vi "PWM.vi"() -> ()   [LabVIEW 2019]
uses:
  <vilib>/myRIO/Instrument Drivers/Onboard IO/PWM/typedefs/PWM Reference.ctl
  <vilib>/myRIO/Common/Instrument Driver Framework/Utilities/typedefs/myRIO Generic Hardware Reference.ctl
  <vilib>/myRIO/Common/Instrument Driver Framework/Utilities/typedefs/Hardware Version Enum.ctl
  <vilib>/myRIO/Common/Instrument Driver Framework/Utilities/typedefs/myRIO v1.0 Reference.ctl
  <vilib>/myRIO/Common/Instrument Driver Framework/Utilities/typedefs/Generic FPGA Reference.ctl
  <vilib>/myRIO/Common/Instrument Driver Framework/myRIO v1.0/PWM/typedefs/PWM Channels Enum.ctl
  <vilib>/myRIO/Instrument Drivers/Onboard IO/PWM/typedefs/PWM Configuration.ctl
  <vilib>/userdefined/High Color/nirio_resource_hc.ctl
  <vilib>/myRIO/Instrument Drivers/Onboard IO/DI Block/typedefs/DI Block Reference.ctl
  <vilib>/myRIO/Common/Instrument Driver Framework/myRIO v1.0/DI Block/typedefs/DI Block Channels List.ctl
  <vilib>/myRIO/Common/Instrument Driver Framework/myRIO v1.0/DI Block/typedefs/DI Block Channels Enum.ctl
  <vilib>/myRIO/Common/Instrument Driver Framework/ELVIS III v1.0/DI Block/vis/ELVIS III v1.1 Open DI (N Samples).vi
  <vilib>/myRIO/Common/Instrument Driver Framework/Utilities/vis/Validate Channels.vi
  <vilib>/myRIO/Common/Instrument Driver Framework/ELVIS III v1.0/Resource Manager/vis/ELVIS III v1.0 Check For Different Banks.vi
  <vilib>/myRIO/Common/Instrument Driver Framework/ELVIS III v1.0/DI Block/vis/ELVIS III v1.0 DI Block Read.vi
  <vilib>/myRIO/Common/Instrument Driver Framework/ELVIS III v1.0/DI Block/vis/ELVIS III v1.0 Close DI Block.vi
  <vilib>/myRIO/Common/Instrument Driver Framework/myRIO v1.0/UART/vis/myRIO v1.0 Close UART.vi
  <vilib>/myRIO/Common/Instrument Driver Framework/Utilities/vis/Sample Rate To Ticks.vi
  <vilib>/myRIO/Common/Instrument Driver Framework/ELVIS III v1.0/DI Block/vis/ELVIS III v1.0 Unreserve DI Block.vi
  <vilib>/myRIO/Common/Instrument Driver Framework/ELVIS III v1.0/Resource Manager/vis/ELVIS III v1.0 Create Configuration List.vi
  <vilib>/myRIO/Common/Instrument Driver Framework/ELVIS III v1.0/DI Block/vis/ELVIS III v1.0 Build MUX Configuration DI Block.vi
  <vilib>/Utility/VariantDataType/GetNumericInfo.vi
  <vilib>/Utility/error.llb/Error Cluster From Error Code.vi
  <vilib>/myRIO/Common/Instrument Driver Framework/ELVIS III v1.0/ELVIS III v1.1 Open.vi
  <vilib>/myRIO/Common/Instrument Driver Framework/ELVIS III v1.0/Resource Manager/vis/ELVIS III v1.0 Reserve Channel List.vi
  <vilib>/myRIO/Common/Instrument Driver Framework/ELVIS III v1.0/Resource Manager/vis/ELVIS III v1.0 Configure IO.vi
  <vilib>/myRIO/Common/Instrument Driver Framework/myRIO v1.0/myRIO v1.0 Close.vi
  <vilib>/myRIO/Common/Instrument Driver Framework/ELVIS III v1.0/DI Block/vis/ELVIS III v1.0 Reserve DI Block.vi
  <vilib>/myRIO/Common/Instrument Driver Framework/ELVIS III v1.0/Resource Manager/vis/ELVIS III v1.0 Configure DMAs.vi
  <vilib>/myRIO/Common/Instrument Driver Framework/myRIO v1.0/Resource Manager/vis/myRIO v1.0 Block Write Configuration.vi
  <vilib>/myRIO/Common/Instrument Driver Framework/ELVIS III v1.0/DI Block/vis/ELVIS III v1.0 DI Block Read Bank B.vi
  <vilib>/myRIO/Common/Instrument Driver Framework/ELVIS III v1.0/DI Block/vis/ELVIS III v1.0 DI Block Read Bank A.vi
  <vilib>/Waveform/DWDTOps.llb/DWDT Boolean Array to Digital.vi
  <vilib>/myRIO/Common/Instrument Driver Framework/ELVIS III v1.0/Resource Manager/vis/ELVIS III v1.0 Unreserve Channel List.vi
  <vilib>/myRIO/Common/Instrument Driver Framework/ELVIS III v1.0/Resource Manager/vis/ELVIS III v1.0 Configure DI Mode.vi
  <vilib>/myRIO/Common/Instrument Driver Framework/Utilities/vis/FPGA Ref Manager.vi
  <vilib>/myRIO/Common/Instrument Driver Framework/ELVIS III v1.0/ELVIS III v1.0 Reset FPGA.vi
  <vilib>/myRIO/Common/Instrument Driver Framework/myRIO v1.0/IRQ/vis/myRIO v1.0 IRQ Info FGV.vi
  <vilib>/myRIO/Common/Instrument Driver Framework/myRIO v1.0/IRQ/vis/myRIO v1.0 Timer IRQ Info FGV.vi
  <vilib>/myRIO/Common/Instrument Driver Framework/myRIO v1.0/IRQ/vis/myRIO v1.0 ISR Agent.vi
  <vilib>/myRIO/Instrument Drivers/Utilities/vis/Reset Index.vi
  <vilib>/myRIO/Common/Instrument Driver Framework/myRIO v1.0/Resource Manager/vis/myRIO v1.0 Block Write Resource Manager.vi
  <vilib>/myRIO/Instrument Drivers/Onboard IO/PWM/vis/myRIO PWM Open.xnode
  <vilib>/myRIO/Instrument Drivers/Onboard IO/DI Block/vis/myRIO DI N Samples Open.xnode
  <vilib>/myRIO/Instrument Drivers/Utilities/Utilities.lvlib
  <vilib>/myRIO/Instrument Drivers/Onboard IO/PWM/PWM.lvlib
  <vilib>/myRIO/Instrument Drivers/Onboard IO/DI Block/DI Block.lvlib
panel:
  out "PWM Signal":digitalwaveform(graph)={"t0"=timestamp(0 s since 1904-01-01), "dt"=0.0001, "Y"={"transitions"=[], "data"=[]}}
  in  "Frequency [Hz]":dbl(knob)=500.0 min=40.0 max=1000.0 scale=40.0..1000.0
  in  "Duty Cycle":dbl(knob)=0.5 min=0.0 max=1.0 scale=0.0..1.0
  in  "?":bool
  # "ELVIS III Control IO"
  # "PWM"
  # "Overview: Generates a PWM signal on Bank A, Channel DIO0 (A/DIO0) with a set duty cycle and frequency and reads the signal on Bank A, Channel DIO1 (A/DIO1).\nInstructions:\n1. Connect A/DIO0 to A/DIO1 to read back the signal on the PWM Signal graph.\n2. Run the VI.\n3. Modify Duty Cycle or Frequency while the VI is running to change the PWM signal."
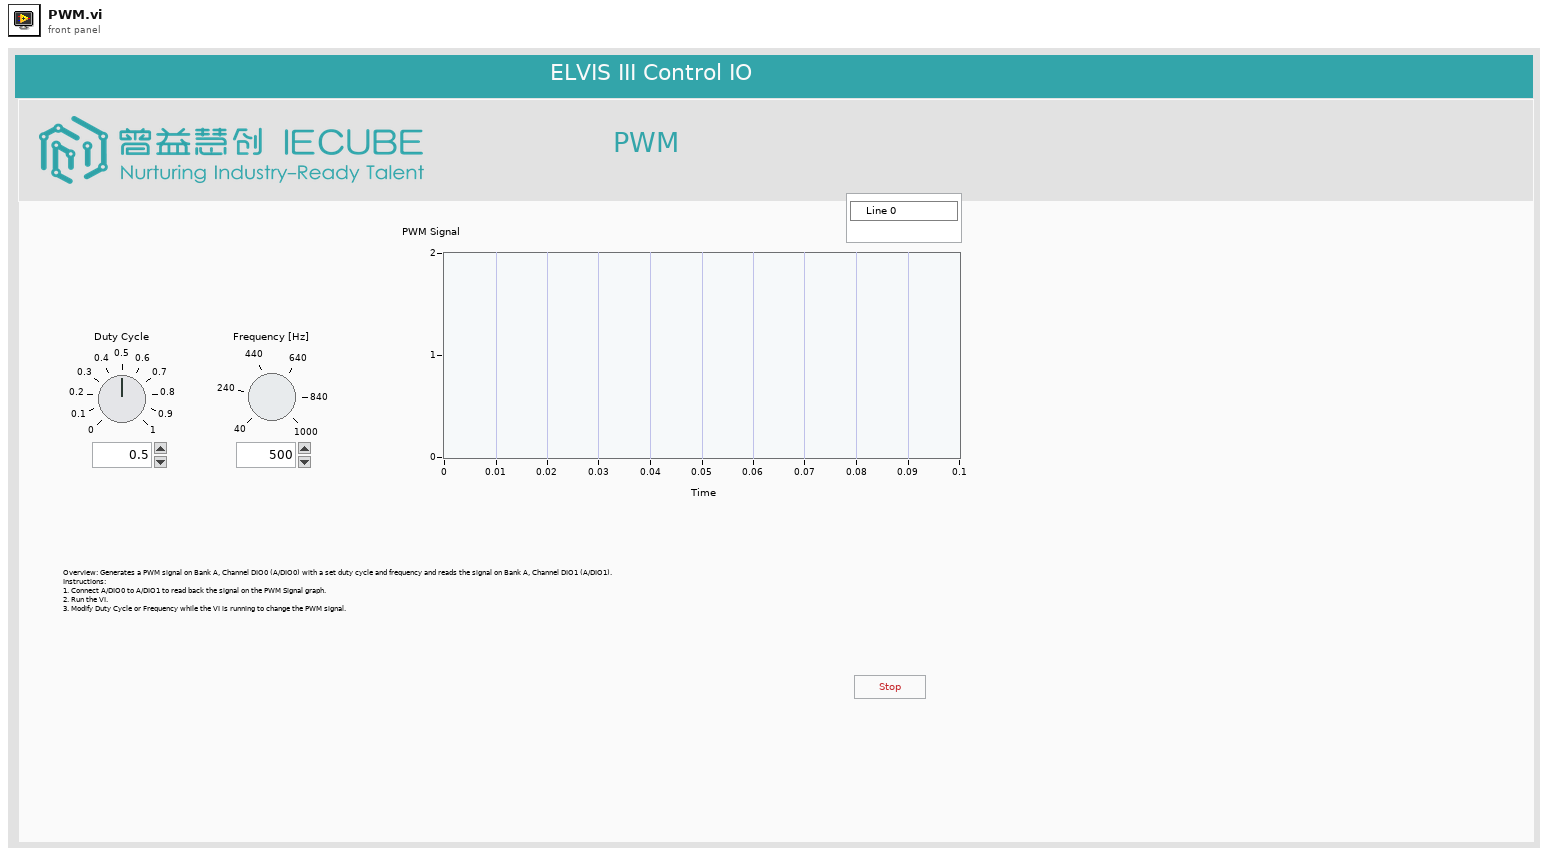
[diagram p1: front panel]
types:
  T1 = typedef "nirio_resource_hc.ctl" = tag
  T2 = typedef "Hardware Version Enum.ctl" = enum16{"Unknown", "myRIO-1900", "myRIO-1950", "roboRIO", "NI ELVIS RIO CM", "ELVIS III"}
  T3 = typedef "PWM.lvlib/PWM Reference.ctl" = cluster{"myRIO Reference":T4, "PWM Channels Enum":T7, "PWM Configuration":T8}
  T4 = typedef "myRIO Generic Hardware Reference.ctl" = cluster{"myRIO Model":T2, "myRIO Hardware Reference":T5}
  T5 = typedef "myRIO v1.0 Reference.ctl" = cluster{"Generic FPGA Reference":T6, "Allow multiple opens":bool}
  T6 = typedef "Generic FPGA Reference.ctl" = refnum<k20>
  T7 = typedef "PWM Channels Enum.ctl" = enum16{"Not Connected", "C/PWM0", "C/PWM1", "A/PWM0", "A/PWM1", "A/PWM2", "A/PWM3", "A/PWM4", "A/PWM5", "A/PWM6", "A/PWM7", "A/PWM8", "A/PWM9", "A/PWM10", "A/PWM11", "A/PWM12", "A/PWM13", "A/PWM14", "A/PWM15", "A/PWM16", "A/PWM17", "A/PWM18", "A/PWM19", "B/PWM0", "B/PWM1", "B/PWM2", "B/PWM3", "B/PWM4", "B/PWM5", "B/PWM6", "B/PWM7", "B/PWM8", "B/PWM9", "B/PWM10", "B/PWM11", "B/PWM12", "B/PWM13", "B/PWM14", "B/PWM15", "B/PWM16", "B/PWM17", "B/PWM18", "B/PWM19", "PWM/PWM0", "PWM/PWM1", "PWM/PWM2", "PWM/PWM3", "PWM/PWM4", "PWM/PWM5", "PWM/PWM6", "PWM/PWM7", "PWM/PWM8", "PWM/PWM9"}
  T8 = typedef "PWM.lvlib/PWM Configuration.ctl" = cluster{"Frequency":dbl, "Duty Cycle":dbl}
  T9 = typedef "DI Block.lvlib/DI Block Reference.ctl" = cluster{"myRIO Reference":T4, "DI (N Samples) Channels List":T10}
  T10 = typedef "DI Block Channels List.ctl" = T11[]
  T11 = typedef "DI Block Channels Enum.ctl" = enum16{"Not Connected", "A/DI0 (N Samples)", "A/DI1 (N Samples)", "A/DI2 (N Samples)", "A/DI3 (N Samples)", "A/DI4 (N Samples)", "A/DI5 (N Samples)", "A/DI6 (N Samples)", "A/DI7 (N Samples)", "A/DI8 (N Samples)", "A/DI9 (N Samples)", "A/DI10 (N Samples)", "A/DI11 (N Samples)", "A/DI12 (N Samples)", "A/DI13 (N Samples)", "A/DI14 (N Samples)", "A/DI15 (N Samples)", "A/DI16 (N Samples)", "A/DI17 (N Samples)", "A/DI18 (N Samples)", "A/DI19 (N Samples)", "B/DI0 (N Samples)", "B/DI1 (N Samples)", "B/DI2 (N Samples)", "B/DI3 (N Samples)", "B/DI4 (N Samples)", "B/DI5 (N Samples)", "B/DI6 (N Samples)", "B/DI7 (N Samples)", "B/DI8 (N Samples)", "B/DI9 (N Samples)", "B/DI10 (N Samples)", "B/DI11 (N Samples)", "B/DI12 (N Samples)", "B/DI13 (N Samples)", "B/DI14 (N Samples)", "B/DI15 (N Samples)", "B/DI16 (N Samples)", "B/DI17 (N Samples)", "B/DI18 (N Samples)", "B/DI19 (N Samples)"}
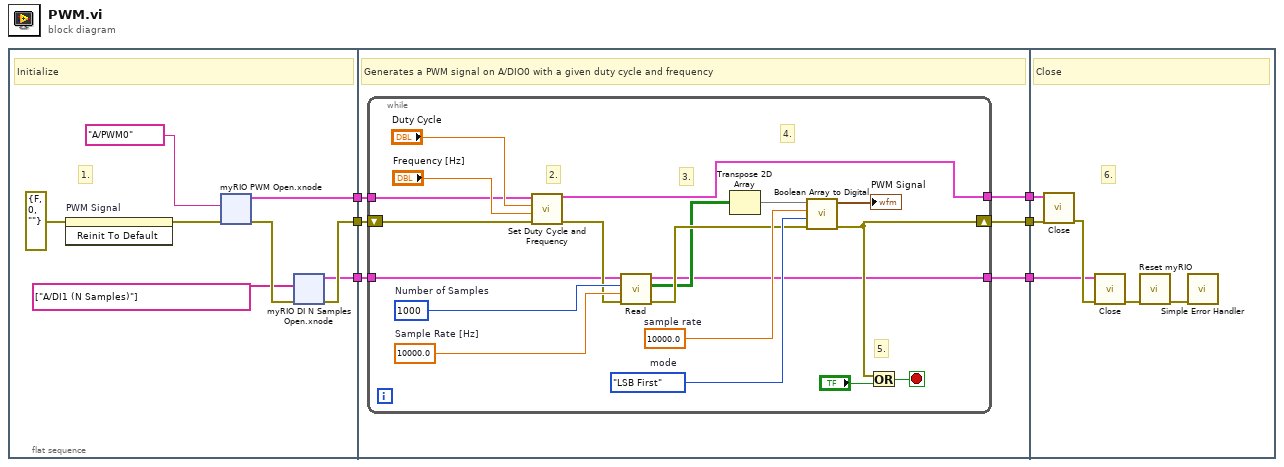
[diagram p0: block diagram]
diagram:
  n1 = flat-sequence {
    tunnel: [w11] -> w5
    tunnel: [w9] -> w4
    tunnel: [w7] -> w3
    tunnel: [w52] -> w6
    tunnel: w5 -> [w51]
    tunnel: w4 -> [w50]
    tunnel: w3 -> [w49]
    tunnel: [w48] -> w2
    tunnel: [w47] -> w1
    tunnel: w6 -> [w76]
    tunnel: w2 -> [w75]
    tunnel: w1 -> [w73]
    frame #0 {
      # "1."
      # "Initialize"
      n2 = invoke on="PWM Signal" class="DigitalGraph (strict)" method="Reinit To Default"(error in=errorcluster {"status"=FALSE, "code"=0, "source"=""} ("Error In")) -> (error out=w13:errorcluster)  [unwired: 2 in, 2 out]
      n3 = xnode "myRIO PWM Open.xnode"("error in (no error)"=w13, "Channel Name"=tag "A/PWM0") -> ("error out"=w12:errorcluster, "PWM Ref Out"=w9:T3)  [unwired: 1 in]
      n4 = xnode "myRIO DI N Samples Open.xnode"("error in (no error)"=w12, "Channel Names"=tag[] ["A/DI1 (N Samples)"]) -> ("error out"=w11:errorcluster, "DI (N Samples) Ref Out"=w7:T9)  [unwired: 1 in]
    }
    frame #1 {
      # "Generates a PWM signal on A/DIO0 with a given duty cycle and frequency"
      n5 = while {
        shift-right: [w66] -> w52
        shift-left: w51 -> [w62]
        tunnel: w50 -> [w61]
        tunnel: w49 -> [w57]
        tunnel: [w54] -> w48
        tunnel: [w53] -> w47
        stop <- w71 stop-if-true
        w59 = 10000.0  # Sample Rate [Hz]
        w60 = u32 1000  # Number of Samples
        w67 = enum16{"LSB First", "MSB First"}."LSB First"  # mode
        w68 = 10000.0  # sample rate
        # "4."
        # "5."
        # "3."
        # "2."
        n6 = call <vilib>:"Set Duty Cycle and Frequency.vi"("error in (no error)"=w62, "Frequency [Hz]"="Frequency [Hz]", "Duty Cycle"="Duty Cycle", "PWM Ref In"=w61) -> ("error out"=w58:errorcluster, "PWM Ref Out"=w54:T3)  [unwired: 5 in]
        n7 = call <vilib>:"Read.vi"("error in (no error)"=w58, "Sample Rate [Hz]"=w59, "Number of Samples"=w60, "DI (N Samples) Ref In"=w57) -> ("error out"=w56:errorcluster, "Values"=w55:bool[][], "DI (N Samples) Ref Out"=w53:T9)  [unwired: 5 in]
        n8 = Transpose 2D Array(2D array=w55) -> (transposed array=w69:bool[][])
        n9 = call-poly <vilib>:"Boolean Array to Digital.vi"("error in (no error)"=w56, "mode"=w67, "sample rate"=w68, "boolean array"=w69) -> ("error out"=w66:errorcluster, "digital waveform"=→"PWM Signal":digitalwaveform)  [unwired: 6 in]
        n10 = Or(x=w66, y="?") -> (x .or. y?=w71:bool)
      }
    }
    frame #2 {
      # "6."
      # "Close"
      n11 = call <vilib>:"Close.vi"("error in (no error)"=w76, "PWM Ref In"=w75) -> ("error out"=w74:errorcluster)  [unwired: 9 in]
      n12 = call <vilib>:"Close.vi"("error in (no error)"=w74, "DI (N Samples) Ref In"=w73) -> ("error out"=w72:errorcluster)  [unwired: 9 in]
      n13 = call <vilib>:"Reset myRIO.vi"("error in (no error)"=w72) -> ("error out"=w77:errorcluster)  [unwired: 10 in]
      n14 = call <vilib>:"Simple Error Handler.vi"("error in (no error)"=w77) -> ()  [unwired: 4 in, 5 out]
    }
  }
